vi "test.VariantBundle.vi"() -> ()   [LabVIEW 2014]
uses:
  Private/Class/meth.Constructor.vi
  Private/Class/meth.Destructor.vi
  GLue.lvlib
panel:
  out "data":cluster{variant, bool}
  out "error out 2":errorcluster
  out "error out":errorcluster
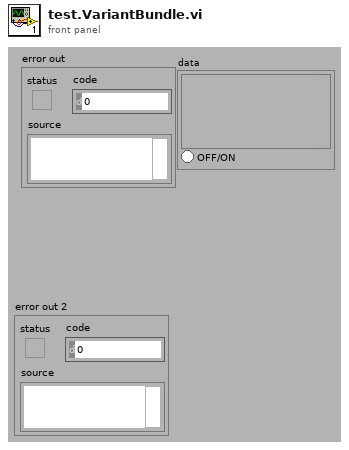
[diagram p1: front panel]
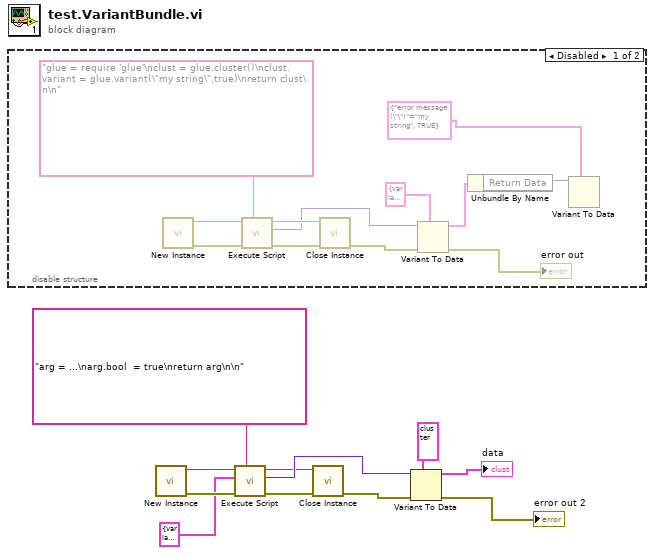
[diagram p0: block diagram]
diagram:
  n1 = disable-structure shown="Disabled" {
    frame Disabled {
      n2 = call "New Instance.vi"() -> ("error out"=w19:errorcluster, "GLue out"=w20:refnum<class "class.GLue.lvclass">)  [unwired: 10 in]
      n3 = call "Execute Script.vi"("Script"="glue = require 'glue'\nclust = glue.cluster()\nclust.variant = glue.variant(\"my string\",true)\nreturn clust\n\n", "error in"=w19, "GLue in"=w20) -> ("error out"=w21:errorcluster, "Return Data"=w17:variant, "GLue out"=w22:refnum<class "class.GLue.lvclass">)  [unwired: 6 in]
      n4 = call "Close Instance.vi"("error in"=w21, "GLue in"=w22) -> ("error out"=w18:errorcluster)  [unwired: 9 in]
      n5 = Variant To Data(error in=w18, type=cluster{"Return Data":variant} {"Return Data"=variant}, Variant=w17) -> (data=w14:cluster{"Return Data":variant}, error out=→"error out":errorcluster)
      n6 = Unbundle By Name(w14) -> ("Return Data"=w13:variant)
      n7 = Variant To Data(type=cluster{"error message (\"\")":string, bool} {"error message (\"\")"="my string", TRUE}, Variant=w13) -> ()  [unwired: 1 in, 2 out]
    }
    frame Enabled {
    }
  }
  n8 = call "New Instance.vi"() -> ("error out"=w8:errorcluster, "GLue out"=w7:refnum<class "class.GLue.lvclass">)  [unwired: 10 in]
  n9 = call "Execute Script.vi"("Script"="arg = ...\narg.bool  = true\nreturn arg\n\n", "error in"=w8, "Argument Data"=cluster{variant} {variant}, "GLue in"=w7) -> ("error out"=w6:errorcluster, "Return Data"=w10:variant, "GLue out"=w5:refnum<class "class.GLue.lvclass">)  [unwired: 5 in]
  n10 = call "Close Instance.vi"("error in"=w6, "GLue in"=w5) -> ("error out"=w9:errorcluster)  [unwired: 9 in]
  n11 = Variant To Data(error in=w9, type=cluster{variant, bool} {variant, FALSE}, Variant=w10) -> (data=→"data":cluster{variant, bool}, error out=→"error out 2":errorcluster)
